vi "NHRCapabilityTest.vi"() -> ()   [LabVIEW 2018]
uses:
  <instrlib>/niScope/Controls/niScope vertical coupling.ctl
  <vilib>/Utility/error.llb/DialogType.ctl
  <instrlib>/niScope/Acquire/Fetch/niScope Multi Fetch WDT.vi
  <vilib>/regexp/Match Regular Expression.xnode
  <instrlib>/NHRDCPowerModule/NHRDCPowerModule/NHRDCPowerModule.lvlib
panel:
  out "x*y":waveform(dbl)[](array[waveform])
  out "wfm info":T1(array[cluster]) {"reserved2" format="%.2f"; "reserved1" format="%.2f"; "offset" format="%^.3e"; "gain" format="%^.3e"; "xIncrement" format="%^.3e"; "relativeInitialX" format="%^.3e"; "absoluteInitialX" format="%^.3e"}
  in  "Sample Rate":dbl=10000000.0 min=1.0 max=10000000.0 format="%_3p S/s"
  out "Scaled Current":dbl[](graph)
  out "Scaled Voltage":dbl[](graph)
  out "maximum voltage slew rate":sgl
  out "maximum current slew rate":sgl
  in  "Hold Time (ms)":sgl=10.0
  in  "Periods/Test":i32=10
  out "NHR On":bool
  in  "V/I Steps":i32=5
  out "Scope On":bool
  in  "Current vertical coupling":T2=1 items=["AC", "DC", "Ground"]
  in  "Current Channel Input Offset":dbl(ring) items=["+25"=25.0, "0"=0.0, "-25"=-25.0]
  out "Current Channel Range":dbl(ring)=10.0 items=["10A"=10.0, "35A"=35.0, "70A"=70.0]
  in  "Voltage vertical coupling":T2=1 items=["AC", "DC", "Ground"]
  in  "Voltage Channel Input Offset":dbl(ring) items=["+500"=500.0, "0"=0.0, "-500"=-500.0]
  out "Voltage Channel Range":dbl(ring)=700.0 items=["200V"=200.0, "700V"=700.0, "1400V"=1400.0]
  in  "Run Test":bool
  in  "Command":u16(ring) items=["Stop All", "Run Test"]
  in  "Test":string(combo)="Voltage"
  in  "Stop VI":bool
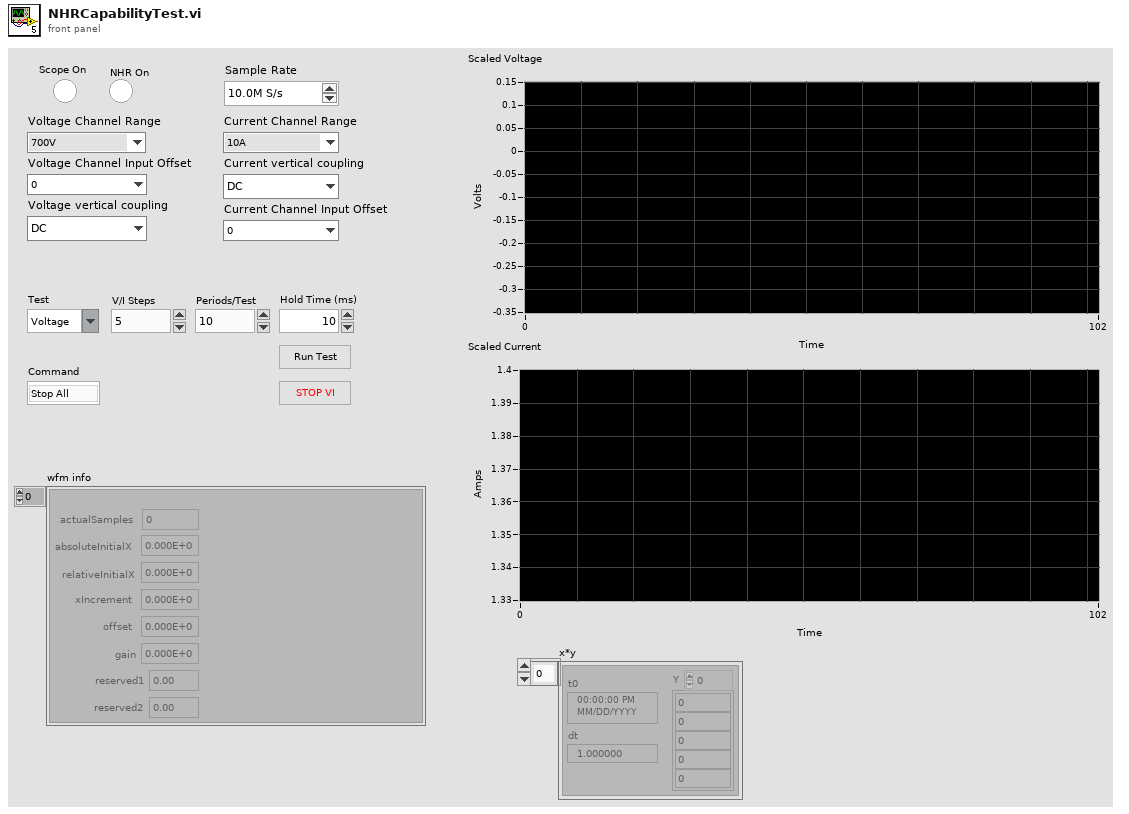
[diagram p1: front panel]
types:
  T1 = cluster{"actualSamples":i32, "absoluteInitialX":dbl, "relativeInitialX":dbl, "xIncrement":dbl, "offset":dbl, "gain":dbl, "reserved1":dbl, "reserved2":dbl}[]
  T2 = typedef "niScope vertical coupling.ctl" = i32
  T3 = enum16{"open", "open or create", "create or replace", "create", "open (read-only)"}
  T4 = typedef "DialogType.ctl" = u16
  T5 = typedef "LVStringsAndValuesArrayTypeDef_DBL.ctl" = cluster{"String":string, "Value":dbl}[]
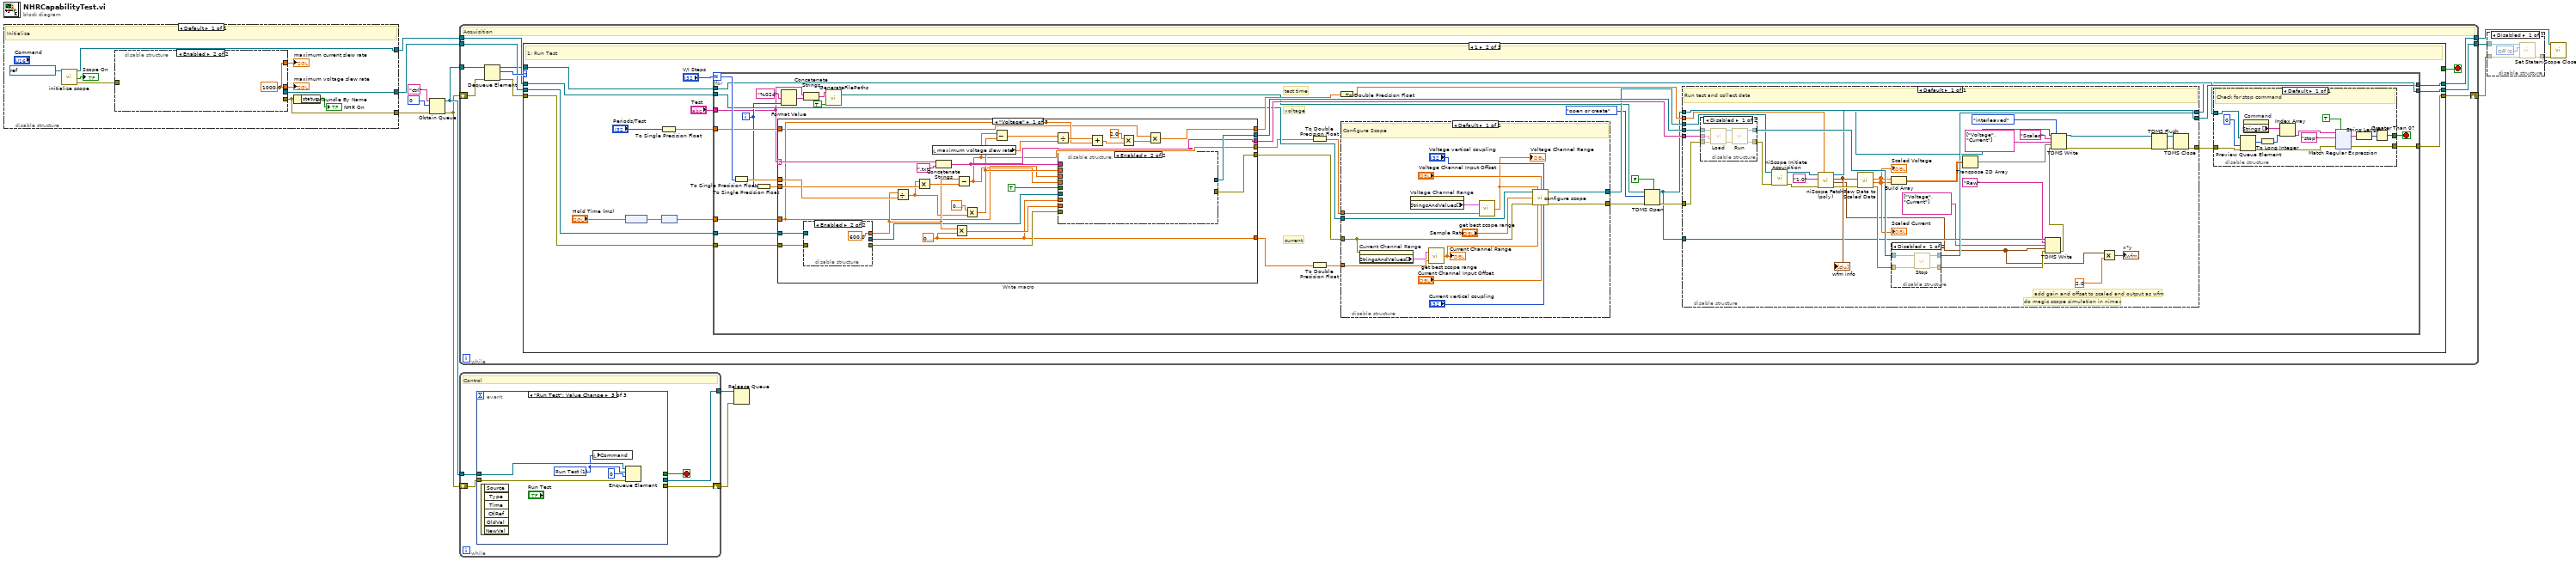
[diagram p0: block diagram]
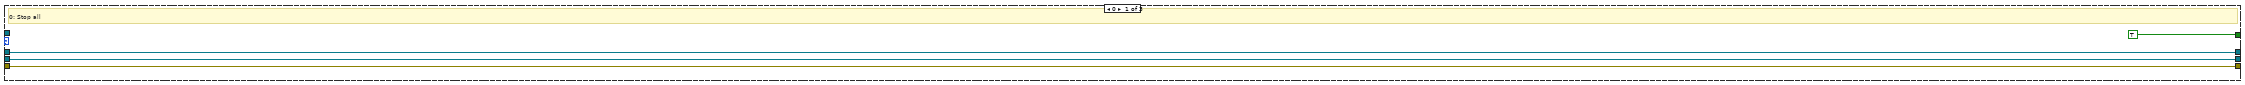
[diagram p3: hidden frame]
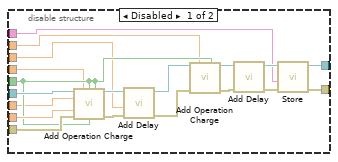
[diagram p6: hidden frame]
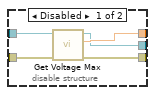
[diagram p7: hidden frame]
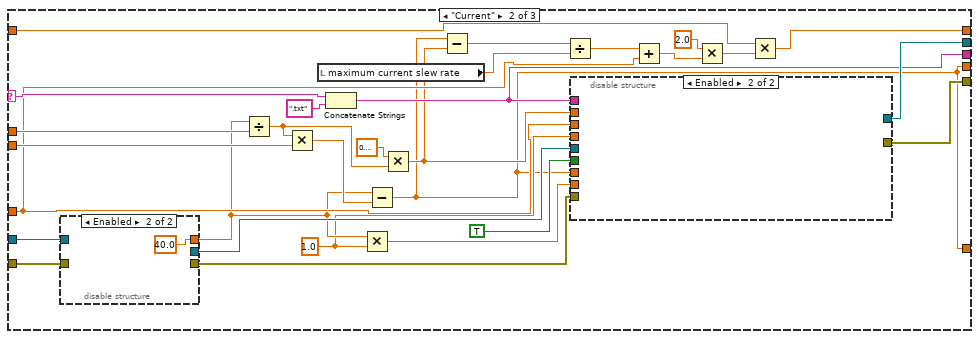
[diagram p8: hidden frame]
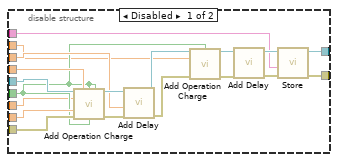
[diagram p9: hidden frame]
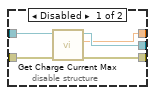
[diagram p10: hidden frame]
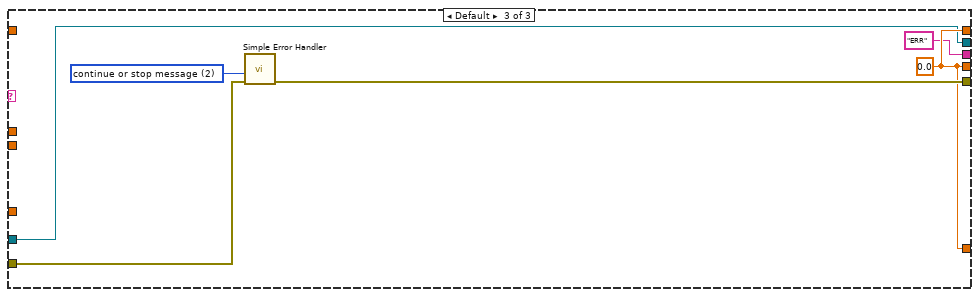
[diagram p11: hidden frame]
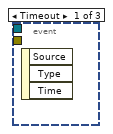
[diagram p13: hidden frame]
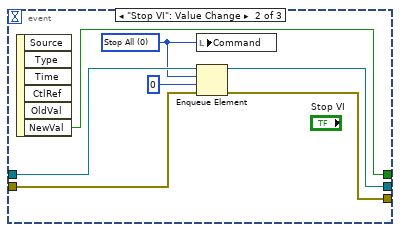
[diagram p14: hidden frame]
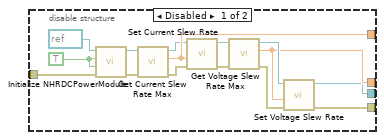
[diagram p15: hidden frame]
diagram:
  w12 = u16 0 items=[""]
  n1 = disable-structure shown="Default" {
    disable-tunnel: [w15] -> w7
    disable-tunnel: [w22] -> w6
    disable-tunnel: [w14] -> w5
    frame Enabled {
      # "Initialize"
      n2 = call "initialize scope.vi"("resource name"=refnum<k15> "oscilloscope") -> ("error out"=w20:errorcluster, "Self-test complete"=→"Scope On":bool, "instrument handle"=w22:refnum<k15>)  [unwired: 3 in, 1 out]
      n3 = disable-structure shown="Enabled" {
        disable-tunnel: w20 -> [w37 _]
        disable-tunnel: [w34 w38] -> w17
        disable-tunnel: [w26 w38] -> w16
        disable-tunnel: [w24 _] -> w15
        disable-tunnel: [w23 _] -> w14
        frame Disabled {
          w35 = TRUE ("id query (Off)")
          n4 = call <instrlib>:"Initialize NHRDCPowerModule.vi"("error in (no error)"=w37, "reset device (Off)"=w35, "id query (Off)"=w35, "resource name"=refnum<visa-resource-name> refnum) -> ("error out"=w32:errorcluster, "instrument handle out"=w31:refnum<visa-resource-name>)  [unwired: 6 in]
          n5 = call <instrlib>:"Get Current Slew Rate Max.vi"("error in (no error)"=w32, "instrument handle"=w31) -> ("error out"=w33:errorcluster, "maximum current slew rate"=w34:sgl, "instrument handle out"=w30:refnum<visa-resource-name>)  [unwired: 7 in]
          n6 = call <instrlib>:"Set Current Slew Rate.vi"("error in (no error)"=w33, "current slew rate (0.0)"=w34, "instrument handle"=w30) -> ("error out"=w28:errorcluster, "instrument handle out"=w29:refnum<visa-resource-name>)  [unwired: 7 in]
          n7 = call <instrlib>:"Get Voltage Slew Rate Max.vi"("error in (no error)"=w28, "instrument handle"=w29) -> ("error out"=w25:errorcluster, "maximum voltage slew rate"=w26:sgl, "instrument handle out"=w27:refnum<visa-resource-name>)  [unwired: 7 in]
          n8 = call <instrlib>:"Set Voltage Slew Rate.vi"("error in (no error)"=w25, "voltage slew rate (0.0)"=w26, "instrument handle"=w27) -> ("error out"=w24:errorcluster, "instrument handle out"=w23:refnum<visa-resource-name>)  [unwired: 7 in]
        }
        frame Enabled {
          w38 = sgl 1000.0 ("maximum current slew rate")
        }
      }
      "maximum current slew rate" <- w17
      "maximum voltage slew rate" <- w16
      n9 = Unbundle By Name(w15) -> ("status"=→"NHR On":bool)
    }
  }
  n10 = Obtain Queue(name (unnamed)="ctrl", element data type=w12, error in (no error)=w7) -> (queue out=w11:refnum<queue>, error out=w10:errorcluster)  [unwired: 2 in, 1 out]
  n11 = while {
    tunnel: w11 -> [w49]
    shift-right: [w39] -> w3
    shift-left: w10 -> [w47]
    tunnel: w6 -> [w44]
    tunnel: w5 -> [w43]
    tunnel: [w42] -> w4
    tunnel: [w40] -> w2
    stop <- w46 stop-if-true
    # "Acquisition"
    n12 = Dequeue Element(queue=w49, error in (no error)=w47) -> (queue out=w41:refnum<queue>, element=w48:u16, error out=w45:errorcluster)  [unwired: 1 in, 1 out]
    n13 = case shown="1" w48 {
      tunnel: [TRUE _ _] -> w46
      tunnel: w45 -> [w50 w60 w408]
      tunnel: w44 -> [w51 w59 w409]
      tunnel: w43 -> [w52 w62 w410]
      tunnel: [w52 w58 w410] -> w42
      tunnel: w41 -> [_ w57 _]
      tunnel: [w51 w55 w409] -> w40
      tunnel: [w50 w56 w408] -> w39
      frame 0 {
        # "0: Stop all"
      }
      frame 1 {
        # "1: Run Test"
        n14 = node("Hold Time (ms)") -> (w64:sgl[unit])
        n15 = To Single Precision Float(number="Periods/Test") -> (single precision float=w61:sgl)
        n16 = node(w64) -> (w63:sgl)
        n17 = for {
          N: "V/I Steps" -> [w102]
          tunnel: w61 -> [w96]
          tunnel: "Test" -> [w70]
          tunnel: w63 -> [w103]
          tunnel: w62 -> [w99]
          tunnel: w60 -> [w88]
          tunnel: w59 -> [w93]
          tunnel: [w76] -> w58
          tunnel: w57 -> [w75]
          tunnel: [w72] -> w56
          tunnel: [w71] -> w55
          i -> [w84]
          stop <- w74 stop-if-true
          # "test time"
          # "current"
          # "voltage"
          n18 = To Single Precision Float(number=w102) -> (single precision float=w101:sgl)
          n19 = To Single Precision Float(number=w84) -> (single precision float=w100:sgl)
          n20 = case "Write macro" shown="\"Voltage\"" w70 {
            selector: w70 -> [w311 w368 _]
            tunnel: w103 -> [w302 w361 _]
            tunnel: w101 -> [w322 w376 _]
            tunnel: w100 -> [w321 w375 _]
            tunnel: w99 -> [w315 w371 w402]
            tunnel: [w309 w366 w402] -> w98
            tunnel: [w308 w365 w405] -> w87
            tunnel: [w307 w364 "ERR"] -> w97
            tunnel: w96 -> [w298 w357 _]
            tunnel: [w297 w354 w404] -> w95
            tunnel: [w296 w348 w404] -> w92
            tunnel: [w295 w348 w404] -> w91
            tunnel: w88 -> [w294 w356 w407]
            frame "Voltage" {
              w296 = sgl 0.1 ("current (0.0)")
              n21 = disable-structure shown="Enabled" {
                disable-tunnel: [w346 sgl 600.0 ("maximum voltage")] -> w319
                disable-tunnel: [w345 _] -> w317
                disable-tunnel: [w344 _] -> w316
                disable-tunnel: w315 -> [w343 _]
                disable-tunnel: w294 -> [w342 _]
                frame Disabled {
                  n22 = call <instrlib>:"Get Voltage Max.vi"("error in (no error)"=w342, "instrument handle"=w343) -> ("error out"=w344:errorcluster, "maximum voltage"=w346:sgl, "instrument handle out"=w345:refnum<visa-resource-name>)  [unwired: 7 in]
                }
                frame Enabled {
                }
              }
              n23 = Divide ("calculate inter-test step")(x=w319, y=w322) -> (x/y=w313:sgl)
              n24 = Multiply(x=w313, y=w321) -> (x*y=w320:sgl)
              n25 = local read "maximum voltage slew rate"() -> (w304:sgl)
              n26 = Concatenate Strings(w311, ".txt" ("string")) -> (w307:string)
              n27 = Multiply ("Get Power")(x=w319, y=w296) -> (x*y=w318:sgl)
              n28 = Subtract ("calculate high value")(x=w319, y=w320) -> (x-y=w295:sgl)
              n29 = Multiply(x=sgl 0.1 ("set low value to 10% of step"), y=w313) -> (x*y=w306:sgl)
              n30 = Subtract ("calculate delta")(x=w295, y=w306) -> (x-y=w305:sgl)
              n31 = Divide ("slew time (s)")(x=w305, y=w304) -> (x/y=w303:sgl)
              n32 = disable-structure shown="Enabled" {
                disable-tunnel: w318 -> [w341 _]
                disable-tunnel: w317 -> [w338 _]
                disable-tunnel: w316 -> [w337 _]
                disable-tunnel: TRUE ("use current (false)") -> [w334 _]
                disable-tunnel: [w329 _] -> w309
                disable-tunnel: [w328 _] -> w308
                disable-tunnel: w307 -> [w327 _]
                disable-tunnel: w306 -> [w326 _]
                disable-tunnel: w302 -> [w325 _]
                disable-tunnel: w296 -> [w324 _]
                disable-tunnel: w295 -> [w323 _]
                frame Disabled {
                  n33 = call <instrlib>:"Add Operation Charge.vi"("instrument handle"=w338, "voltage (0.0)"=w323, "use current (false)"=w334, "use voltage (false)"=w334, "current (0.0)"=w324, "power (0.0)"=w341, "error in (no error)"=w337, "use power (false)"=w334) -> ("instrument handle out"=w340:refnum<visa-resource-name>, "error out"=w339:errorcluster)  [unwired: 6 in]
                  n34 = call <instrlib>:"Add Delay.vi"("error in (no error)"=w339, "delay (0.0)"=w325, "instrument handle"=w340) -> ("error out"=w335:errorcluster, "instrument handle out"=w336:refnum<visa-resource-name>)  [unwired: 7 in]
                  n35 = call <instrlib>:"Add Operation Charge.vi"("instrument handle"=w336, "voltage (0.0)"=w326, "use voltage (false)"=w334, "error in (no error)"=w335) -> ("instrument handle out"=w332:refnum<visa-resource-name>, "error out"=w333:errorcluster)  [unwired: 10 in]
                  n36 = call <instrlib>:"Add Delay.vi"("error in (no error)"=w333, "instrument handle"=w332) -> ("error out"=w330:errorcluster, "instrument handle out"=w331:refnum<visa-resource-name>)  [unwired: 8 in]
                  n37 = call <instrlib>:"Store.vi"("error in (no error)"=w330, "path (\"\")"=w327, "instrument handle"=w331) -> ("error out"=w328:errorcluster, "instrument handle out"=w329:refnum<visa-resource-name>)  [unwired: 7 in]
                }
                frame Enabled {
                }
              }
              n38 = Add(x=w303, y=w302) -> (x+y=w301:sgl)
              n39 = Multiply ("single wave period")(x=sgl 2.0, y=w301) -> (x*y=w299:sgl)
              n40 = Multiply ("test period")(x=w298, y=w299) -> (x*y=w297:sgl)
            }
            frame "Current" {
              w351 = sgl 1.0 ("voltage (0.0)")
              n41 = disable-structure shown="Enabled" {
                disable-tunnel: [w400 _] -> w373
                disable-tunnel: [w399 _] -> w372
                disable-tunnel: w371 -> [w398 _]
                disable-tunnel: w356 -> [w397 _]
                disable-tunnel: [w396 sgl 40.0 ("charge current max")] -> w353
                frame Disabled {
                  n42 = call <instrlib>:"Get Charge Current Max.vi"("error in (no error)"=w397, "instrument handle"=w398) -> ("error out"=w399:errorcluster, "charge current max"=w396:sgl, "instrument handle out"=w400:refnum<visa-resource-name>)  [unwired: 7 in]
                }
                frame Enabled {
                }
              }
              n43 = Divide ("calculate inter-test step")(x=w353, y=w376) -> (x/y=w370:sgl)
              n44 = Multiply(x=w370, y=w375) -> (x*y=w374:sgl)
              n45 = local read "maximum current slew rate"() -> (w355:sgl)
              n46 = Concatenate Strings(w368, ".txt" ("string")) -> (w364:string)
              n47 = Multiply ("Get Power")(x=w353, y=w351) -> (x*y=w352:sgl)
              n48 = Subtract ("calculate high value")(x=w353, y=w374) -> (x-y=w348:sgl)
              n49 = Multiply(x=sgl 0.1 ("set low value to 10% of step"), y=w370) -> (x*y=w349:sgl)
              n50 = Subtract ("calculate delta")(x=w348, y=w349) -> (x-y=w363:sgl)
              n51 = Divide ("slew time (s)")(x=w363, y=w355) -> (x/y=w362:sgl)
              n52 = disable-structure shown="Enabled" {
                disable-tunnel: w373 -> [w393 _]
                disable-tunnel: w372 -> [w392 _]
                disable-tunnel: [w385 _] -> w366
                disable-tunnel: [w384 _] -> w365
                disable-tunnel: w364 -> [w383 _]
                disable-tunnel: w361 -> [w382 _]
                disable-tunnel: w352 -> [w381 _]
                disable-tunnel: w351 -> [w380 _]
                disable-tunnel: TRUE ("use current (false)") -> [w379 _]
                disable-tunnel: w349 -> [w378 _]
                disable-tunnel: w348 -> [w377 _]
                frame Disabled {
                  n53 = call <instrlib>:"Add Operation Charge.vi"("instrument handle"=w393, "voltage (0.0)"=w380, "use current (false)"=w379, "use voltage (false)"=w379, "current (0.0)"=w377, "power (0.0)"=w381, "error in (no error)"=w392, "use power (false)"=w379) -> ("instrument handle out"=w395:refnum<visa-resource-name>, "error out"=w394:errorcluster)  [unwired: 6 in]
                  n54 = call <instrlib>:"Add Delay.vi"("error in (no error)"=w394, "delay (0.0)"=w382, "instrument handle"=w395) -> ("error out"=w390:errorcluster, "instrument handle out"=w391:refnum<visa-resource-name>)  [unwired: 7 in]
                  n55 = call <instrlib>:"Add Operation Charge.vi"("instrument handle"=w391, "use current (false)"=w379, "current (0.0)"=w378, "error in (no error)"=w390) -> ("instrument handle out"=w388:refnum<visa-resource-name>, "error out"=w389:errorcluster)  [unwired: 10 in]
                  n56 = call <instrlib>:"Add Delay.vi"("error in (no error)"=w389, "instrument handle"=w388) -> ("error out"=w386:errorcluster, "instrument handle out"=w387:refnum<visa-resource-name>)  [unwired: 8 in]
                  n57 = call <instrlib>:"Store.vi"("error in (no error)"=w386, "path (\"\")"=w383, "instrument handle"=w387) -> ("error out"=w384:errorcluster, "instrument handle out"=w385:refnum<visa-resource-name>)  [unwired: 7 in]
                }
                frame Enabled {
                }
              }
              n58 = Add(x=w362, y=w361) -> (x+y=w360:sgl)
              n59 = Multiply ("single wave period")(x=sgl 2.0, y=w360) -> (x*y=w358:sgl)
              n60 = Multiply ("test period")(x=w357, y=w358) -> (x*y=w354:sgl)
            }
            frame Default {
              w404 = sgl 0.0
              w406 = T4 2 items=["no dialog", "OK message", "continue or stop message", "OK message + warnings", "continue/stop + warnings"] ("type of dialog (OK msg:1)")
              n61 = call <vilib>:"Simple Error Handler.vi"("type of dialog (OK msg:1)"=w406, "error in (no error)"=w407) -> ("error out"=w405:errorcluster)  [unwired: 3 in, 4 out]
            }
          }
          n62 = Format Value(format string="%02d", value (0)=w84) -> (output string=w83:string)  [unwired: 1 in]
          n63 = Concatenate Strings(w70, w83) -> (w82:string)
          n64 = call "GenerateFilePaths.vi"("Logfile? (F)"=TRUE, "Device Name"=w82) -> ("Path"=w79:path)  [unwired: 3 in]
          n65 = To Double Precision Float(number=w91) -> (double precision float=w89:dbl)
          n66 = To Double Precision Float(number=w92) -> (double precision float=w90:dbl)
          n67 = To Double Precision Float(number=w95) -> (double precision float=w94:dbl)
          n68 = disable-structure shown="Default" {
            disable-tunnel: w87 -> [w283]
            disable-tunnel: w93 -> [w293]
            disable-tunnel: w90 -> [w288]
            disable-tunnel: w89 -> [w287]
            disable-tunnel: [w281] -> w77
            disable-tunnel: [w280] -> w86
            frame Enabled {
              # "Configure Scope"
              n69 = property on="Current Channel Range" class="Ring (strict)"(error in=w283) -> ("StringsAndValues[]"=w282:T5)  [unwired: 1 in, 2 out]
              n70 = property on="Voltage Channel Range" class="Ring (strict)"() -> ("StringsAndValues[]"=w285:T5)  [unwired: 2 in, 2 out]
              n71 = call "get best scope range.vi"("Set point"=w288, "Range Strings and Values"=w282) -> ("Best Range"=w284:dbl)
              "Current Channel Range" <- w284
              n72 = call "get best scope range.vi"("Set point"=w287, "Range Strings and Values"=w285) -> ("Best Range"=w286:dbl)
              "Voltage Channel Range" <- w286
              n73 = call "configure scope.vi"("instrument handle"=w293, "Voltage Channel Range"=w286, "Voltage Channel Input Offset"="Voltage Channel Input Offset", "Voltage vertical coupling"="Voltage vertical coupling", "Sample Rate"="Sample Rate", "error in"=w283, "Current Channel Range"=w284, "Current Channel Input Offset"="Current Channel Input Offset", "Current vertical coupling"="Current vertical coupling") -> ("instrument handle out"=w280:refnum<k15>, "error out"=w281:errorcluster)  [unwired: 3 in, 2 out]
            }
          }
          n74 = TDMS Open(5:FALSE ("create index file? (T)"), 8:w77, 10:T3."open or create" ("operation (0:open)"), 11:w79) -> (0:w78:errorcluster, 3:w68:refnum<k34>)  [unwired: 3 in]
          n75 = disable-structure shown="Default" {
            disable-tunnel: w98 -> [w267]
            disable-tunnel: w97 -> [w266]
            disable-tunnel: w94 -> [w260]
            disable-tunnel: w78 -> [w257]
            disable-tunnel: w86 -> [w256]
            disable-tunnel: w68 -> [w241]
            disable-tunnel: [w247] -> w76
            disable-tunnel: [w246] -> w73
            disable-tunnel: [w245] -> w71
            disable-tunnel: w68 -> [w239]
            frame Enabled {
              # "do magic scope simulation in nimax"
              # "add gain and offset to scaled and output as wfm"
              # "Run test and collect data"
              n76 = disable-structure shown="Disabled" {
                disable-tunnel: w267 -> [w278 _]
                disable-tunnel: w266 -> [w277 _]
                disable-tunnel: [w275 _] -> w265
                disable-tunnel: [w273 _] -> w261
                disable-tunnel: w257 -> [w272 _]
                frame Disabled {
                  n77 = call <instrlib>:"Load.vi"("error in (no error)"=w272, "path (\"\")"=w277, "instrument handle"=w278) -> ("error out"=w274:errorcluster, "instrument handle out"=w276:refnum<visa-resource-name>)  [unwired: 7 in]
                  n78 = call <instrlib>:"Run.vi"("error in (no error)"=w274, "instrument handle"=w276) -> ("error out"=w273:errorcluster, "instrument handle out"=w275:refnum<visa-resource-name>)  [unwired: 8 in]
                }
                frame Enabled {
                }
              }
              n79 = call <instrlib>:"niScope Initiate Acquisition.vi"("instrument handle"=w256, "error in"=w261) -> ("instrument handle out"=w263:refnum<k15>, "error out"=w262:errorcluster)  [unwired: 12 in]
              n80 = call-poly <instrlib>:"niScope Fetch (poly).vi"("timeout"=w260, "error in"=w262, "channels"="1,0", "instrument handle"=w263) -> ("error out"=w259:errorcluster, "wfm"=w234:waveform(dbl)[], "wfm info"=w240:T1, "instrument handle out"=w245:refnum<k15>)  [unwired: 4 in]
              "wfm info" <- w240
              n81 = call "Raw Data to Scaled Data.vi"("error In"=w259, "Wvf Info"=w240) -> ("error out"=w258:errorcluster, "Scaled Current"=w244:dbl[], "Scaled Voltage"=w254:dbl[])  [unwired: 5 in, 2 out]
              "Scaled Voltage" <- w254
              "Scaled Current" <- w244
              n82 = Build Array(w254, w244) -> (w253:dbl[][])
              n83 = disable-structure shown="Disabled" {
                disable-tunnel: w265 -> [w271 _]
                disable-tunnel: w258 -> [w270 _]
                disable-tunnel: [w269 _] -> w236
                disable-tunnel: [w268 _] -> w247
                frame Disabled {
                  n84 = call <instrlib>:"Stop.vi"("error in (no error)"=w270, "instrument handle"=w271) -> ("error out"=w269:errorcluster, "instrument handle out"=w268:refnum<visa-resource-name>)  [unwired: 8 in]
                }
                frame Enabled {
                }
              }
              n85 = Transpose 2D Array(2D array=w253) -> (transposed array=w243:dbl[][])
              n86 = TDMS Write(0:w239, 5:"Raw" ("group name in (Untitled)"), 7:string[] ["Voltage", "Current"] ("channel name(s) in (Untitled)"), 9:w234, 11:w236) -> (15:w235:errorcluster)  [unwired: 1 in, 3 out]
              n87 = TDMS Write(0:w241, 1:enum16{"decimated", "interleaved"}."interleaved" ("data layout (0:decimated)"), 5:"Scaled" ("group name in (Untitled)"), 7:string[] ["Voltage", "Current"] ("channel name(s) in (Untitled)"), 9:w243, 11:w235) -> (4:w250:refnum<k34>, 15:w251:errorcluster)  [unwired: 2 out]
              n88 = Multiply(x=w234, y=2.0) -> (x*y=→"x*y":waveform(dbl)[])
              n89 = TDMS Flush(4:w251, 7:w250) -> (0:w248:errorcluster, 3:w249:refnum<k34>)
              n90 = TDMS Close(8:w248, 11:w249) -> (0:w246:errorcluster)  [unwired: 1 out]
            }
          }
          n91 = disable-structure shown="Default" {
            disable-tunnel: w75 -> [w117]
            disable-tunnel: [w107] -> w74
            disable-tunnel: w73 -> [w106]
            disable-tunnel: [w104] -> w72
            frame Enabled {
              # "Check for stop command"
              n92 = Preview Queue Element(queue=w117, timeout in ms (-1)=0, error in (no error)=w106) -> (element=w114:u16, error out=w105:errorcluster)  [unwired: 2 out]
              n93 = property on="Command" class="Ring (strict)"() -> ("Strings []"=w115:string[])  [unwired: 2 in, 2 out]
              n94 = To Long Integer(number=w114) -> (32bit integer=w113:i32)
              n95 = Index Array(array=w115, index=w113) -> (element=w111:string)
              n96 = xnode "Match Regular Expression"("input string"=w111, "regular expression"="stop", "error in"=w105, "ignore case? (F)"=TRUE) -> ("whole match"=w109:string, "error out"=w104:errorcluster)  [unwired: 2 in, 3 out]
              n97 = String Length(string=w109) -> (length=w108:i32)
              n98 = Greater Than 0?(x=w108) -> (x > 0?=w107:bool)
            }
          }
        }
      }
      frame Default {
      }
    }
  }
  n99 = while {
    tunnel: w11 -> [w414]
    tunnel: [w412] -> w9
    shift-right: [w411] -> w8
    shift-left: w10 -> [w413]
    stop <- w415 stop-if-true
    # "Control"
    n100 = event shown="[2] \"Run Test\": Value Change" {
      selector: _ -> [_ _ _]
      dyn-events: _ -> [_ _ _]
      timeout: _ -> [_ _ _]
      tunnel: [_ w422 _] -> w415
      tunnel: w414 -> [_ w421 w425]
      tunnel: w413 -> [_ w419 w424]
      tunnel: [_ w418 _] -> w412
      tunnel: [_ w417 _] -> w411
      event Timeout {
        n101 = event-data() -> ()  [unwired: 1 in, 3 out]
      }
      event "Stop VI": Value Change {
        w416 = u16 0 items=["Stop All"] ("Command")
        n102 = event-data() -> ("NewVal"=w422:bool)  [unwired: 1 in, 5 out]
        n103 = local write "Command"(w416) -> ()
        n104 = Enqueue Element(queue=w421, element=w416, timeout in ms (-1)=0, error in (no error)=w419) -> (queue out=w418:refnum<queue>, error out=w417:errorcluster)  [unwired: 1 out]
      }
      event "Run Test": Value Change {
        w423 = u16 1 items=["Stop All", "Run Test"] ("Command")
        n105 = event-data() -> ()  [unwired: 1 in, 6 out]
        n106 = local write "Command"(w423) -> ()
        n107 = Enqueue Element(queue=w425, element=w423, timeout in ms (-1)=0, error in (no error)=w424) -> ()  [unwired: 3 out]
      }
    }
  }
  n108 = Release Queue(queue=w9, error in (no error)=w8) -> ()  [unwired: 1 in, 3 out]
  n109 = disable-structure shown="Disabled" {
    disable-tunnel: w4 -> [w430 _]
    disable-tunnel: w3 -> [w429 _]
    disable-tunnel: [w428 _] -> w1
    frame Disabled {
      w427 = 0 items=["Off", "Stand By", "Charge", "Discharge", "Battery Emulation"] ("operating state (Off)")
      n110 = call <instrlib>:"Set State.vi"("instrument handle"=w430, "operating state (Off)"=w427, "error in (no error)"=w429) -> ("error out"=w428:errorcluster)  [unwired: 11 in, 1 out]
    }
    frame Enabled {
    }
  }
  n111 = call <instrlib>:"niScope Close.vi"("instrument handle"=w2, "error in"=w1) -> ()  [unwired: 13 in, 1 out]
